vi "refresh_token.vi"(6 "timeout (ms)":i32=10000, 7 "IP address":string, 8 "error in (no error)":errorcluster, 10 "token cluster in":T1, 11 "client handle":T2) -> (0 "error out":errorcluster, 2 "token cluster":T1, 3 "client handle out":T2)   [LabVIEW 2018]
uses:
  <vilib>/httpClient/ClientHandle.ctl
  <vilib>/httpClient/POSTBuffer.vi
  <vilib>/httpClient/LabVIEWHTTPClient.lvlib
panel:
  out "headers":string
  out "code":string
  out "msg":string
  out "reponse":string
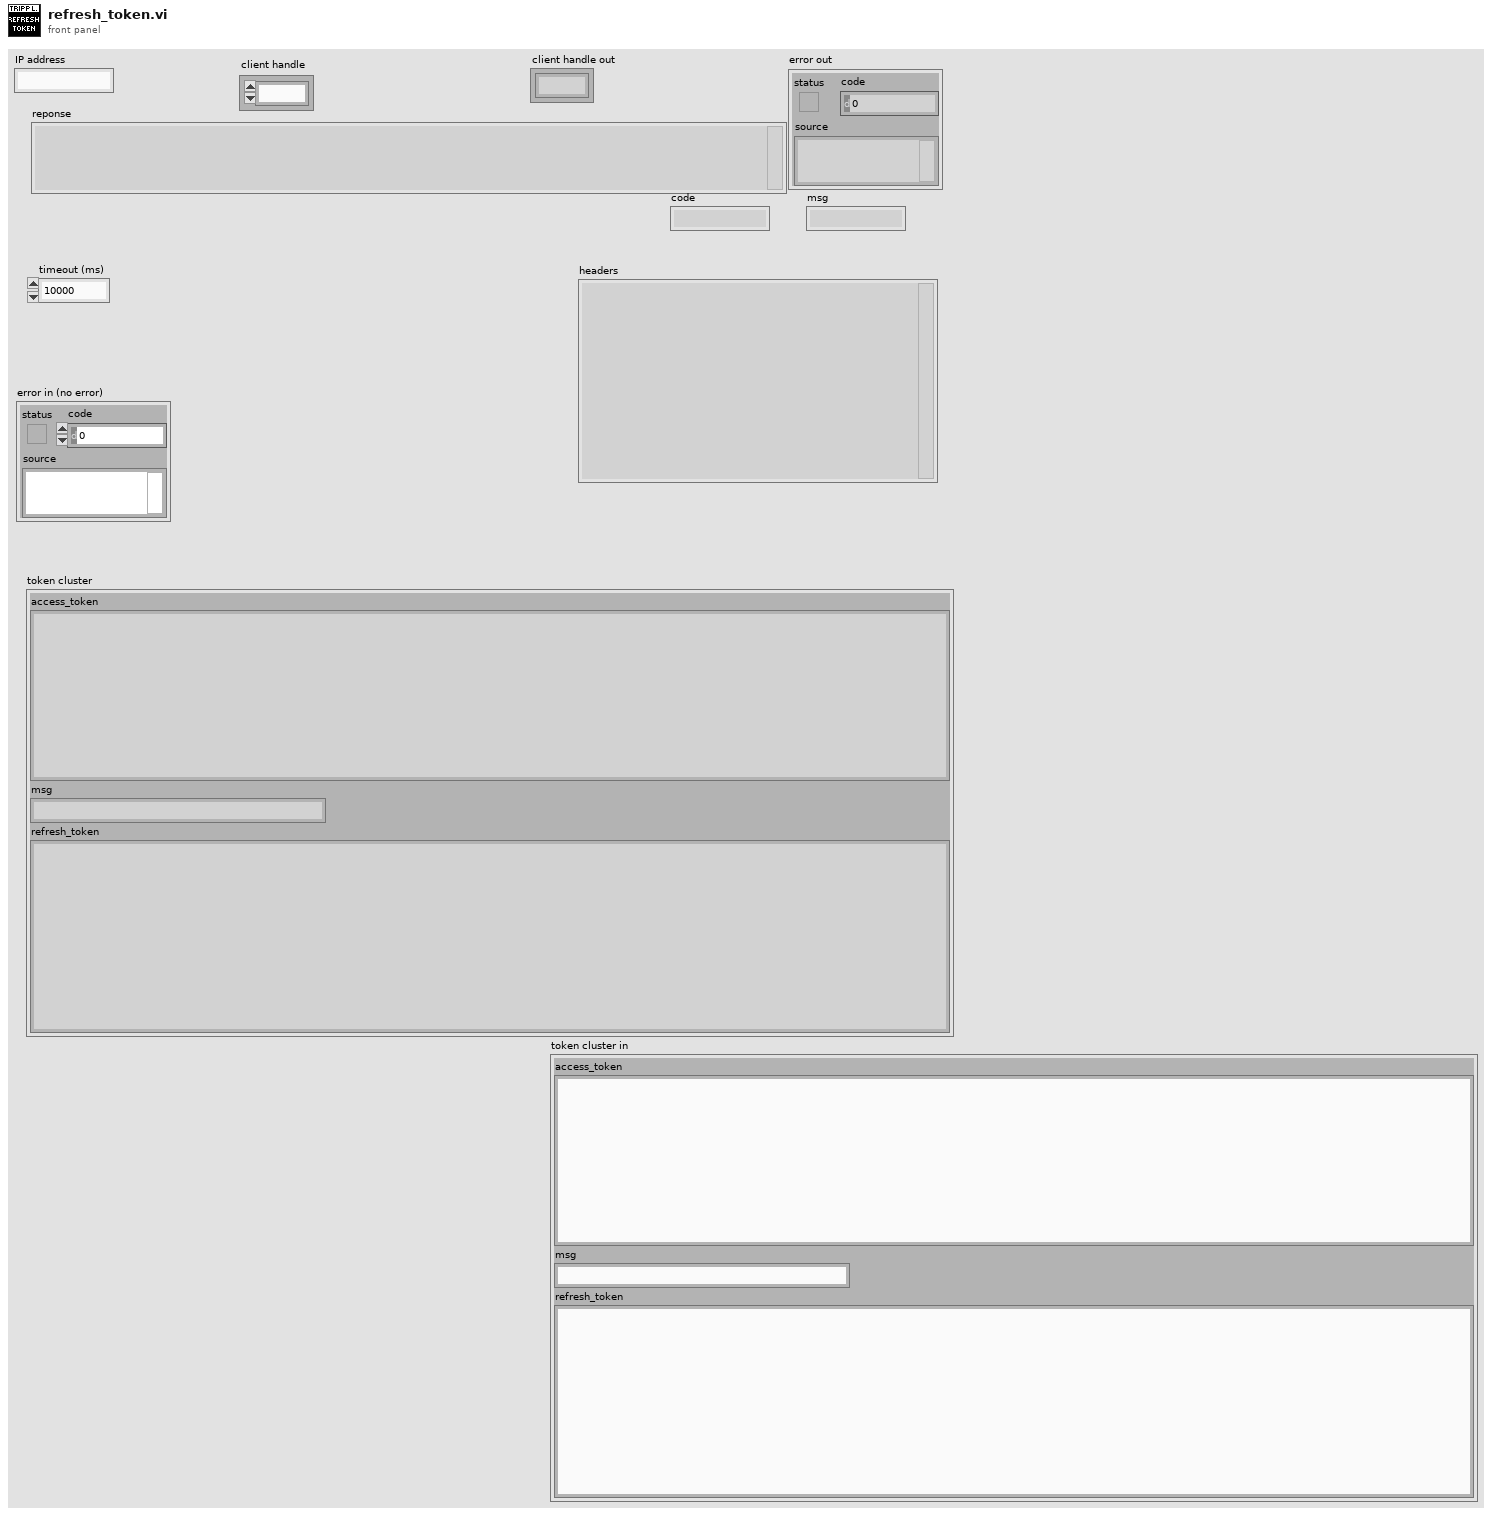
[diagram p1: front panel]
types:
  T1 = cluster{"access_token":string, "msg":string, "refresh_token":string}
  T2 = typedef "LabVIEWHTTPClient.lvlib/ClientHandle.ctl" = refnum<k1>
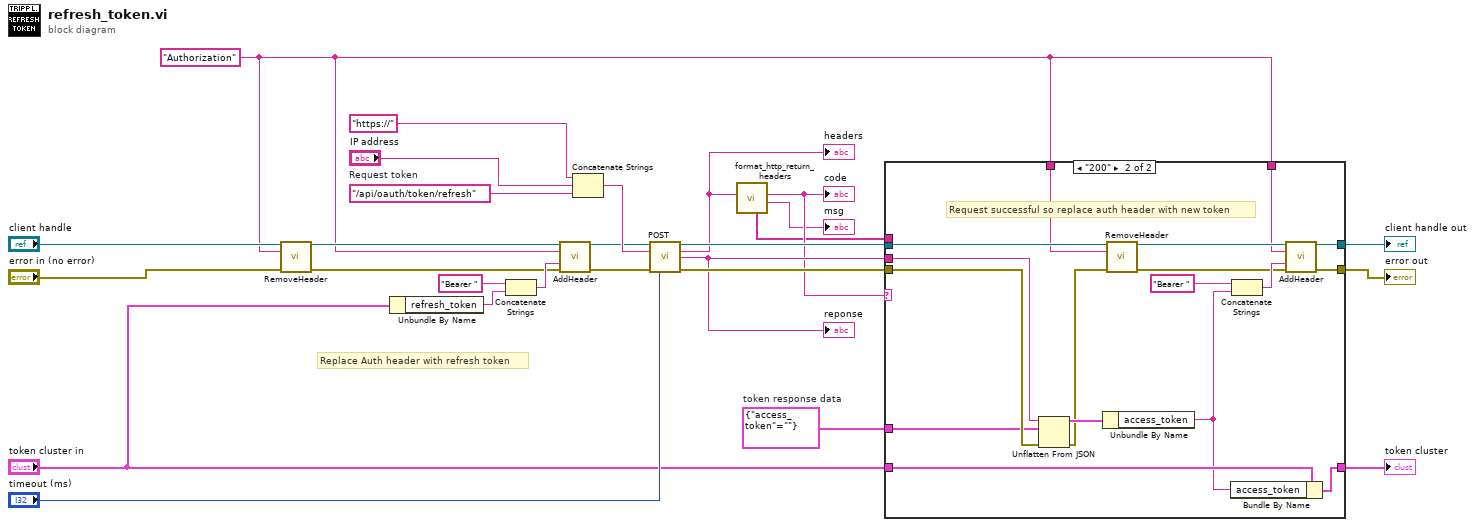
[diagram p0: block diagram]
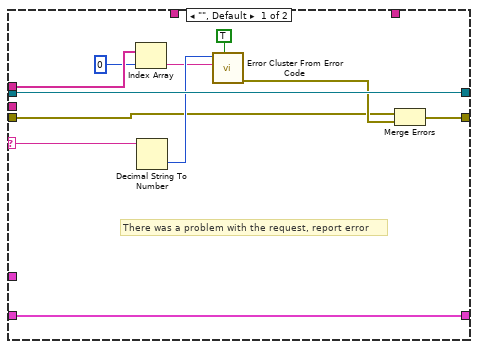
[diagram p2: hidden frame]
diagram:
  w1 = "Authorization" ("value")
  w16 = cluster{"access_token":string} {"access_token"=""}  # token response data
  w23 = "/api/oauth/token/refresh"  # Request token
  # "Replace Auth header with refresh token"
  n1 = call <vilib>:"RemoveHeader.vi"("client handle"="client handle", "header"=w1, "error in (no error)"="error in (no error)") -> ("client handle out"=w9:T2, "error out"=w8:errorcluster)  [unwired: 11 in]
  n2 = Unbundle By Name("token cluster in") -> ("refresh_token"=w6:string)
  n3 = Concatenate Strings("Bearer " ("value"), w6) -> (w10:string)
  n4 = call <vilib>:"AddHeader.vi"("client handle"=w9, "header"=w1, "value"=w10, "error in (no error)"=w8) -> ("client handle out"=w5:T2, "error out"=w7:errorcluster)  [unwired: 10 in]
  n5 = Concatenate Strings("https://", "IP address", w23) -> (w27:string)
  n6 = call-poly <vilib>:"POST.vi"("client handle"=w5, "url"=w27, "error in (no error)"=w7, "timeout (10000)"="timeout (ms)") -> ("client handle out"=w24:T2, "headers"=w18:string, "body"=w25:string, "error out"=w26:errorcluster)  [unwired: 8 in]
  "reponse" <- w25
  "headers" <- w18
  n7 = call "format_http_return_headers.vi"("headers in"=w18) -> ("msg"=→"msg":string, "status code"=w17:string, "headers array"=w14:string[])  [unwired: 8 in]
  "code" <- w17
  n8 = case shown="\"200\"" w17 {
    selector: w17 -> [w35 _]
    tunnel: w26 -> [w30 w55]
    tunnel: w25 -> [_ w54]
    tunnel: w24 -> [w38 w43]
    tunnel: [w29 w51] -> w20
    tunnel: [w38 w50] -> w19
    tunnel: w16 -> [_ w49]
    tunnel: [w28 w45] -> w12
    tunnel: w14 -> [w34 _]
    tunnel: "token cluster in" -> [w28 w47]
    tunnel: w1 -> [_ w40]
    tunnel: w1 -> [_ w39]
    frame "", Default {
      # "There was a problem with the request, report error"
      n9 = Index Array(array=w34, index=0) -> (element=w32:string)
      n10 = Decimal String To Number(string=w35) -> (number=w36:i32)  [unwired: 2 in, 1 out]
      n11 = call <vilib>:"Error Cluster From Error Code.vi"("show call chain? (False)"=TRUE, "error message (\"\")"=w32, "error code (0)"=w36) -> ("error out"=w31:errorcluster)  [unwired: 6 in]
      n12 = Merge Errors(w30, w31) -> (w29:errorcluster)
    }
    frame "200" {
      # "Request successful so replace auth header with new token"
      n13 = Unflatten From JSON(JSON string=w54, type and defaults=w49, error in (no error)=w55) -> (value=w48:cluster{"access_token":string}, error out=w44:errorcluster)  [unwired: 4 in]
      n14 = Unbundle By Name(w48) -> ("access_token"=w46:string)
      n15 = call <vilib>:"RemoveHeader.vi"("client handle"=w43, "header"=w40, "error in (no error)"=w44) -> ("client handle out"=w42:T2, "error out"=w41:errorcluster)  [unwired: 11 in]
      n16 = Bundle By Name(cluster=w47, "access_token"=w46) -> (w45:T1)
      n17 = Concatenate Strings("Bearer " ("value"), w46) -> (w52:string)
      n18 = call <vilib>:"AddHeader.vi"("client handle"=w42, "header"=w39, "value"=w52, "error in (no error)"=w41) -> ("client handle out"=w50:T2, "error out"=w51:errorcluster)  [unwired: 10 in]
    }
  }
  "error out" <- w20
  "client handle out" <- w19
  "token cluster" <- w12
